vi "JSON Flatten Configuration.vi"(8 "error in (no error)":errorcluster, 10 "file version":T1, 11 "configuration":T2={"plugins"=[{"name"="Plugin", "components"=[], "cycle timing"={"priority"=10000, "decimation"=1, "offset"=0}, "threads"=[], "transfer groups"=[{"name"="Group", "direction"=enum."Tx", "cycle timing"={"priority"=100, "decimation"=1, "offset"=0}, "thread index"=255, "settings"=[], "transfers"=[{"name"="Transfer", "byte order"=enum."big-endian", "settings"=[], "channels"=[{"string offset"=0, "name"="Channel", "units"="V", "engine data type"=enum."DBL", "string data type"=enum."DBL", "settings"=[]}]}], "timeout behavior"=enum."Increment Late Count", "convert buffers"=FALSE}], "settings"=[]}]}) -> (0 "error out":errorcluster, 2 "actual file version":T1, 3 "configuration json":string)   [LabVIEW 2017, in "DSF Core.lvlib" / "Configuration Session.lvclass"]
uses:
  Configuration Session.lvclass
  Typedefs/DSF Engine Framework Configuration.ctl
  Typedefs/DSF Engine Plugin Configuration.ctl
  Typedefs/DSF Timing Info.ctl
  Typedefs/DSF Engine Plugin Thread Configuration.ctl
  Typedefs/DSF Settings Info.ctl
  Typedefs/DSF Engine Transfer Group Configuration.ctl
  Typedefs/DSF Direction.ctl
  Typedefs/DSF Engine Transfer Configuration.ctl
  Typedefs/DSF Byte Order.ctl
  Typedefs/DSF Engine Channel Configuration.ctl
  Typedefs/DSF Data Type.ctl
  Typedefs/DSF Timeout Behavior.ctl
  Typedefs/DSF Version Info.ctl
  DSF Core.lvlib
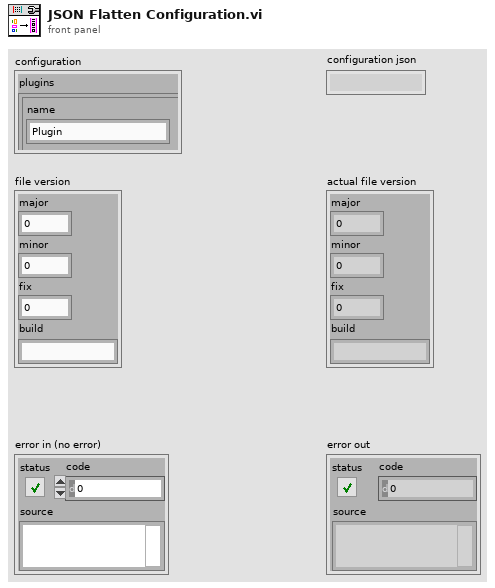
[diagram p1: front panel]
types:
  T1 = typedef "DSF Core.lvlib/DSF Version Info.ctl" = cluster{"major":u32, "minor":u32, "fix":u32, "build":string}
  T2 = typedef "DSF Core.lvlib/DSF Engine Framework Configuration.ctl" = cluster{"plugins":T3[]}
  T3 = typedef "DSF Core.lvlib/DSF Engine Plugin Configuration.ctl" = cluster{"name":string, "components":string[], "cycle timing":T4, "threads":T5[], "transfer groups":T7[], "settings":T6}
  T4 = typedef "DSF Core.lvlib/DSF Timing Info.ctl" = cluster{"priority":u64, "decimation":u64, "offset":u64}
  T5 = typedef "DSF Core.lvlib/DSF Engine Plugin Thread Configuration.ctl" = cluster{"processor":i32, "priority offset":i16, "settings":T6}
  T6 = typedef "DSF Core.lvlib/DSF Settings Info.ctl" = cluster{"component":string, "name":string, "values":cluster{"key":string, "value":string}[]}[]
  T7 = typedef "DSF Core.lvlib/DSF Engine Transfer Group Configuration.ctl" = cluster{"name":string, "direction":T8, "cycle timing":T4, "thread index":u8, "settings":T6, "transfers":T9[], "timeout behavior":T13, "convert buffers":bool}
  T8 = typedef "DSF Core.lvlib/DSF Direction.ctl" = enum8{"Tx", "Rx"}
  T9 = typedef "DSF Core.lvlib/DSF Engine Transfer Configuration.ctl" = cluster{"name":string, "byte order":T10, "settings":T6, "channels":T11[]}
  T10 = typedef "DSF Core.lvlib/DSF Byte Order.ctl" = enum8{"big-endian", "little-endian"}
  T11 = typedef "DSF Core.lvlib/DSF Engine Channel Configuration.ctl" = cluster{"string offset":u64, "name":string, "units":string, "engine data type":T12, "string data type":T12, "settings":T6}
  T12 = typedef "DSF Core.lvlib/DSF Data Type.ctl" = enum8{"Bool", "SGL", "DBL", "I8", "I16", "I32", "I64", "U8", "U16", "U32", "U64"}
  T13 = typedef "DSF Core.lvlib/DSF Timeout Behavior.ctl" = enum8{"Increment Late Count", "Throw Error"}
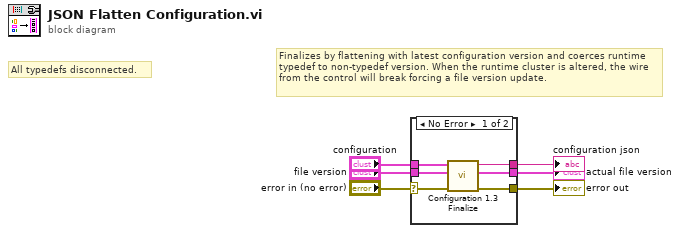
[diagram p0: block diagram]
diagram:
  # "Finalizes by flattening with latest configuration version and coerces runtime typedef to non-typedef version. When the runtime cluster is altered, the wire from the control will break forcing a file version update."
  # "All typedefs disconnected."
  n1 = case shown="No Error" "error in (no error)" {
    selector: "error in (no error)" -> [w11 w13]
    tunnel: [w8 w13] -> w6
    tunnel: "configuration" -> [w12 _]
    tunnel: [w10 _] -> w3
    tunnel: [w9 _] -> w2
    tunnel: "file version" -> [w7 _]
    frame No Error {
      n2 = call "Configuration 1.3 Finalize.vi"("error in (no error)"=w11, "file version (x.y)"=w7, "configuration 1.3"=w12) -> ("error out"=w8:errorcluster, "final file version"=w9:T1, "configuration json"=w10:string)  [unwired: 6 in]
    }
    frame Error {
    }
  }
  "configuration json" <- w3
  "error out" <- w6
  "actual file version" <- w2
